vi "Config Updated.vi"(8 "error in (no error)":errorcluster, 11 "SerialResource in":refnum<class "SerialResource.lvclass">) -> (0 "error out":errorcluster, 3 "SerialResource out":refnum<class "SerialResource.lvclass">)   [LabVIEW 2020, in "PicoG-Core.lvlib" / "SerialResource.lvclass"]
uses:
  SerialResource.lvclass
  SerialResource.lvclass/SerialResource.ctl
  Resource/Resource.lvclass
  C:/dev/picoG/PicoG/PicoG-Core/Resource/Resource.lvclass
  C:/dev/picoG/PicoG/PicoG-Core/SerialResource/SerialResource.lvclass
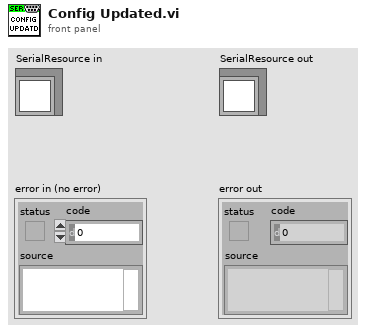
[diagram p1: front panel]
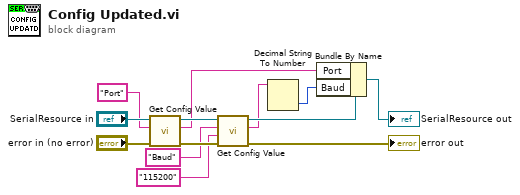
[diagram p0: block diagram]
diagram:
  n1 = call "Get Config Value.vi"("error in (no error)"="error in (no error)", "Name"="Port", "Resource in"="SerialResource in") -> ("error out"=w11:errorcluster, "Value"=w4:string, "Resource out"=w12:refnum<class "SerialResource.lvclass">)  [unwired: 5 in, 1 out]
  n2 = call "Get Config Value.vi"("error in (no error)"=w11, "Default"="115200" ("Name"), "Name"="Baud", "Resource in"=w12) -> ("error out"=→"error out":errorcluster, "Value"=w2:string, "Resource out"=w5:refnum<class "SerialResource.lvclass">)  [unwired: 4 in, 1 out]
  n3 = Decimal String To Number(string=w2) -> (number=w1:i32)  [unwired: 2 in, 1 out]
  n4 = Bundle By Name(cluster=w5, "Port"=w4, "Baud"=w1) -> (→"SerialResource out":refnum<class "SerialResource.lvclass">)
